vi "gaussian correlation time with pause.vi"() -> ()   [LabVIEW 2014]
uses:
  <vilib>/userdefined/High Color/IMAQdx.ctl
  <vilib>/Utility/file.llb/Write To Spreadsheet File (DBL).vi
  <vilib>/vision/driver/NI_Vision_Acquisition_Software.lvlib
panel:
  in  "Stimulus Duration (frames)":dbl
  in  "Pause Duration (frames)":dbl
  in  "Correlation Time (s)":dbl
  in  "Start Recording":bool
  in  "Max Voltage":dbl
  in  "Min Voltage":dbl
  in  "Frames":i32
  in  "Sigma":dbl
  in  "Offset Voltage":dbl
  out "Error":string
  out "Save Directory":path
  out "Buffer Number Out":u32
  out "Image":T1(plugin-control)
  in  "stop":bool
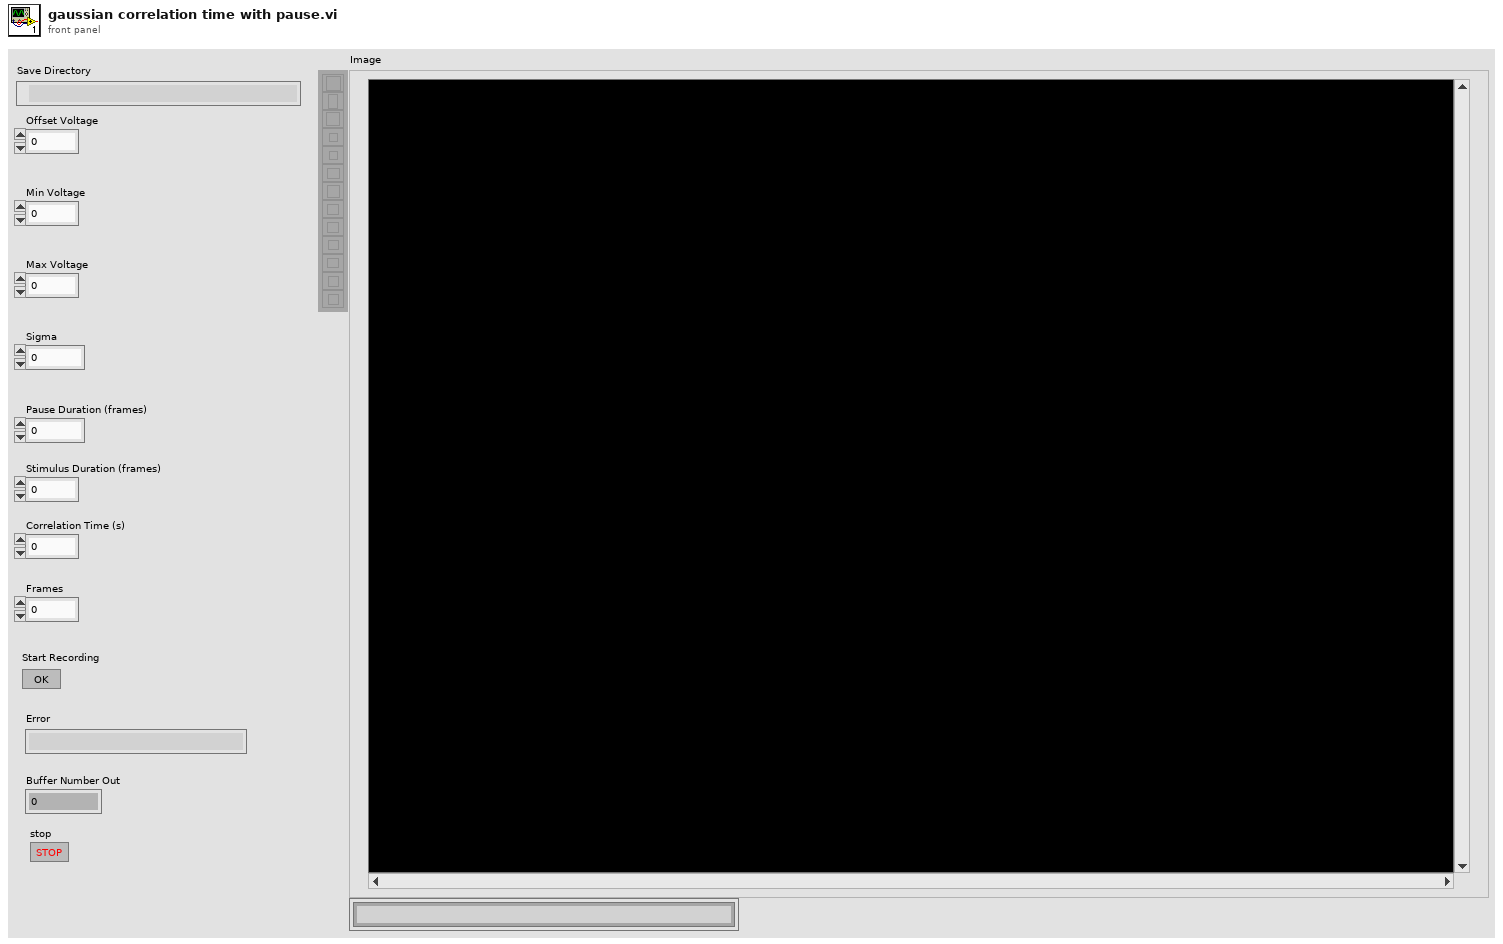
[diagram p1: front panel]
types:
  T1 = typedef "IMAQ Image.ctl" = refnum<image>
  T2 = typedef "IMAQdx.ctl" = refnum<k21>
  T3 = cluster{"Rows Per Strip":i32, "Photometric":i32, "Compression Type":i32}
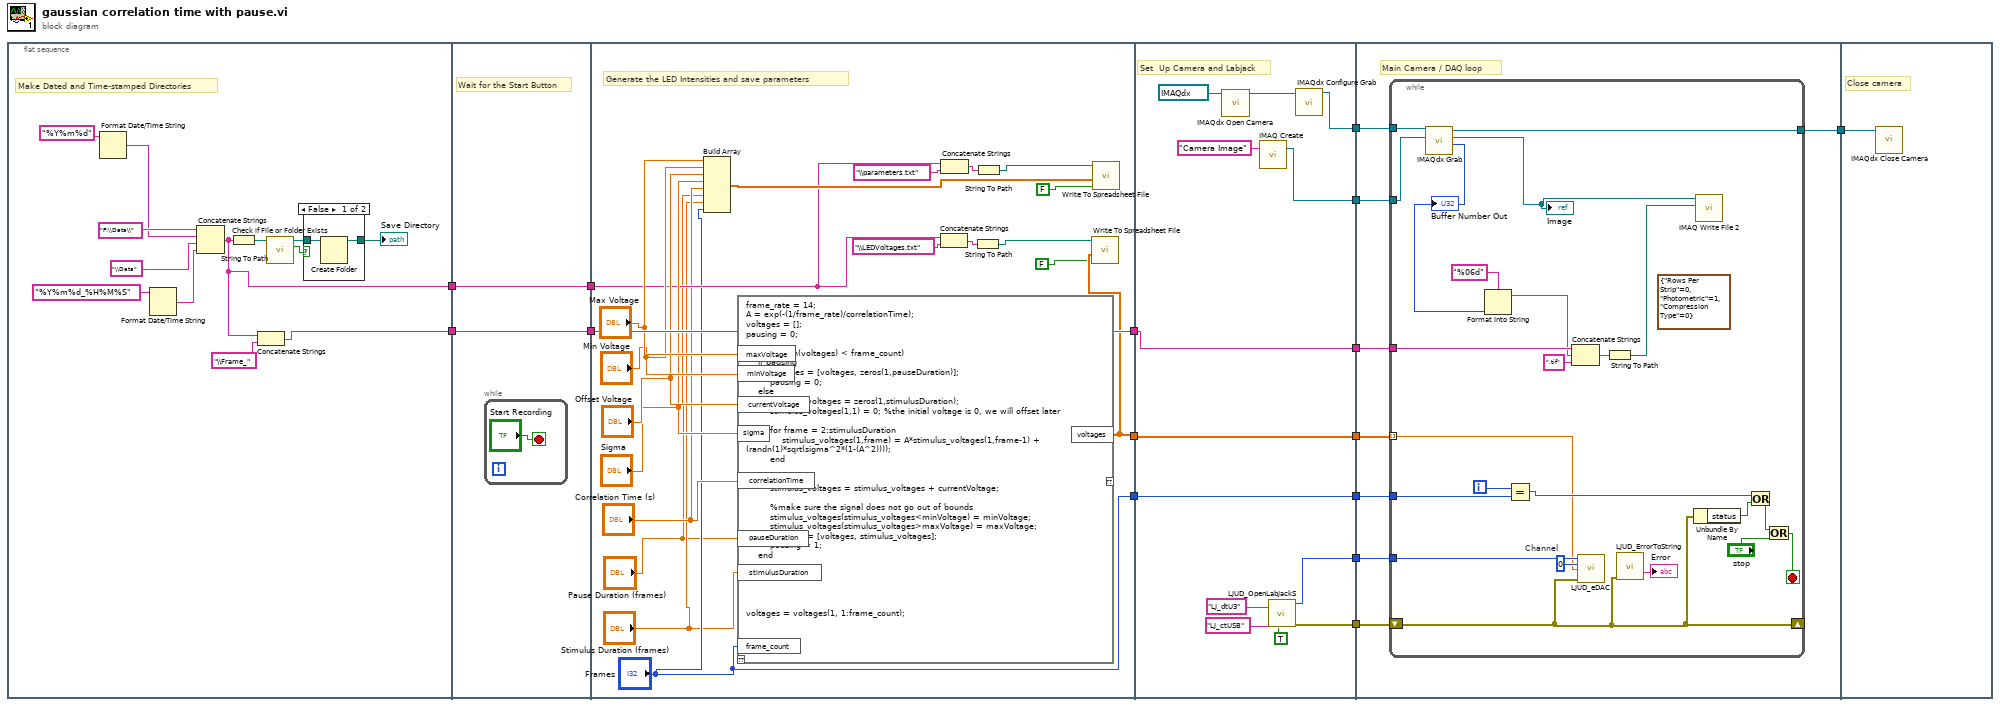
[diagram p0: block diagram]
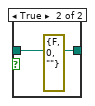
[diagram p2: hidden frame]
diagram:
  n1 = flat-sequence {
    tunnel: [w18] -> w4
    tunnel: [w16] -> w2
    tunnel: w4 -> [w33]
    tunnel: [w33] -> w3
    tunnel: w2 -> [w32]
    tunnel: [w32] -> w1
    tunnel: w3 -> [w52]
    tunnel: [w52] -> w9
    tunnel: [w50] -> w7
    tunnel: ["Frames"] -> w6
    tunnel: w1 -> [w39]
    tunnel: w9 -> [w62]
    tunnel: [w64] -> w15
    tunnel: [w63] -> w14
    tunnel: [w62] -> w13
    tunnel: [w58] -> w11
    tunnel: [w57] -> w10
    tunnel: [w56] -> w8
    tunnel: w7 -> [w56]
    tunnel: w6 -> [w55]
    tunnel: [w55] -> w5
    tunnel: w15 -> [w75]
    tunnel: w14 -> [w74]
    tunnel: w13 -> [w73]
    tunnel: [w72] -> w12
    tunnel: w11 -> [w71]
    tunnel: w10 -> [w70]
    tunnel: w8 -> [w69]
    tunnel: w5 -> [w68]
    tunnel: w12 -> [w99]
    frame #0 {
      # "Make Dated and Time-stamped Directories"
      n2 = Format Date/Time String(time format string (%c)="%Y%m%d") -> (date/time string=w19:string)  [unwired: 2 in]
      n3 = Format Date/Time String(time format string (%c)="%Y%m%d_%H%M%S") -> (date/time string=w23:string)  [unwired: 2 in]
      n4 = Concatenate Strings("F:\\Data\\", w19, "\\Data", w23) -> (w16:string)
      n5 = String To Path(string=w16) -> (path=w22:path)
      n6 = Concatenate Strings(w16, "\\Frame_") -> (w18:string)
      n7 = call <vilib>:"Check if File or Folder Exists.vi"("path"=w22) -> ("file or folder exists?"=w27:bool, "dup path"=w26:path)  [unwired: 8 in, 1 out]
      n8 = case shown="False" w27 {
        tunnel: [w29 w31] -> w21
        tunnel: w26 -> [w30 w31]
        frame False {
          n9 = Create Folder(path (use dialog)=w30) -> (created path=w29:path)  [unwired: 2 in, 2 out]
        }
        frame True {
          (unwired) errorcluster {"status"=FALSE, "code"=0, "source"=""} ("error out")
        }
      }
      "Save Directory" <- w21
    }
    frame #1 {
      # "Wait for the Start Button"
      n10 = while {
        stop <- "Start Recording" stop-if-true
      }
    }
    frame #2 {
      # "Generate the LED Intensities and save parameters"
      n11 = Build Array("Max Voltage", "Min Voltage", "Offset Voltage", "Sigma", "Correlation Time (s)", "Pause Duration (frames)", "Stimulus Duration (frames)", "Frames") -> (w40:dbl[])
      n12 = script code="frame_rate = 14;\nA = exp(-(1/frame_rate)/correlationTime);\nvoltages = [];\npausing = 0;\n\nwhile (length(voltages) < frame_count)\n    if pausing\n        voltages = [voltages, zeros(1,pauseDuration)];\n        pausing = 0;\n    else\n        stimulus_voltages = zeros(1,stimulusDuration);\n        stimulus_voltages(1,1) = 0; %the initial voltage is 0, we will offset later\n\n        for frame = 2:stimulusDuration\n            stimulus_voltages(1,frame) = A*stimulus_voltages(1,frame-1) + (randn(1)*sqrt(sigma^2*(1-(A^2))));\n        end\n\n        %offset\n        stimulus_voltages = stimulus_voltages + currentVoltage;\n\n        %make sure the signal does not go out of bounds\n        stimulus_voltages(stimulus_voltages<minVoltage) = minVoltage;\n        stimulus_voltages(stimulus_voltages>maxVoltage) = maxVoltage;\n        voltages = [voltages, stimulus_voltages];\n        pausing = 1;\n    end\n\nend\n\n\n\nvoltages = voltages(1, 1:frame_count);"("currentVoltage"="Offset Voltage", "frame_count"="Frames", "sigma"="Sigma", "minVoltage"="Min Voltage", "maxVoltage"="Max Voltage", "correlationTime"="Correlation Time (s)", "pauseDuration"="Pause Duration (frames)", "stimulusDuration"="Stimulus Duration (frames)") -> ("voltages"=w50:dbl[])  [unwired: 1 in, 1 out]
      n13 = Concatenate Strings(w39, "\\LEDVoltages.txt") -> (w54:string)
      n14 = Concatenate Strings(w39, "\\parameters.txt") -> (w44:string)
      n15 = String To Path(string=w54) -> (path=w53:path)
      n16 = String To Path(string=w44) -> (path=w43:path)
      n17 = call-poly <vilib>:"Write To Spreadsheet File.vi"("append to file? (new file:F)"=FALSE, "1D data"=w50, "file path (dialog if empty)"=w53) -> ()  [unwired: 5 in, 1 out]
      n18 = call-poly <vilib>:"Write To Spreadsheet File.vi"("append to file? (new file:F)"=FALSE, "1D data"=w40, "file path (dialog if empty)"=w43) -> ()  [unwired: 5 in, 1 out]
    }
    frame #3 {
      # "Set  Up Camera and Labjack"
      n19 = call <vilib>:"IMAQdx Open Camera.vi"("Session In"=T2 "cam0") -> ("Session Out"=w66:T2)  [unwired: 9 in, 1 out]
      n20 = call "IMAQ Create"("Image Name"="Camera Image") -> ("New Image"=w63:T1)  [unwired: 4 in, 1 out]
      n21 = call "LJUD_OpenLabJackS.vi"("FirstFound"=TRUE, "ConnectionType"="LJ_ctUSB", "DeviceType"="LJ_dtU3") -> ("error out"=w57:errorcluster, "Handle"=w58:i32)  [unwired: 6 in, 1 out]
      n22 = call <vilib>:"IMAQdx Configure Grab.vi"("Session In"=w66) -> ("Session Out"=w64:T2)  [unwired: 9 in, 1 out]
    }
    frame #4 {
      # "Main Camera / DAQ loop"
      n23 = while {
        tunnel: w75 -> [w98]
        tunnel: [w97] -> w72
        tunnel: w74 -> [w96]
        tunnel: w73 -> [w94]
        tunnel: w71 -> [w87]
        shift-right: [w84] -> _
        shift-left: w70 -> [w84]
        tunnel: w69 -> [w76] mode=indexing
        tunnel: w68 -> [w77]
        i -> [w78]
        stop <- w86 stop-if-true
        w83 = 0  # Channel
        (unwired) T3 {"Rows Per Strip"=0, "Photometric"=1, "Compression Type"=0} ("TIFF Options")
        n24 = call <vilib>:"IMAQdx Grab.vi"("Image In"=w96, "Session In"=w98) -> ("Buffer Number Out"=w90:u32, "Image Out"=w95:T1, "Session Out"=w97:T2)  [unwired: 6 in, 1 out]
        "Image" <- w95
        "Buffer Number Out" <- w90
        n25 = Format Into String(format string="%06d" ("string"), w90) -> (resulting string=w89:string)  [unwired: 2 in, 1 out]
        n26 = Equal?(x=w78, y=w77) -> (x = y?=w80:bool)
        n27 = Concatenate Strings(w94, w89, ".tif" ("string")) -> (w92:string)
        n28 = call "LJUD_eDAC.vi"("Handle In"=w87, "Channel"=w83, "Voltage"=w76, "error in"=w84) -> ()  [unwired: 10 in, 2 out]
        n29 = String To Path(string=w92) -> (path=w91:path)
        n30 = call "LJUD_ErrorToString.vi"("error in"=w84) -> ("String"=→"Error":string)  [unwired: 10 in]
        n31 = Unbundle By Name(w84) -> ("status"=w81:bool)
        n32 = call-poly "IMAQ Write File 2"("File Path"=w91, "Image"=w95) -> ()  [unwired: 8 in, 2 out]
        n33 = Or(x=w80, y=w81) -> (x .or. y?=w79:bool)
        n34 = Or(x=w79, y="stop") -> (x .or. y?=w86:bool)
      }
    }
    frame #5 {
      # "Close camera"
      n35 = call <vilib>:"IMAQdx Close Camera.vi"("Session In"=w99) -> ()  [unwired: 10 in, 1 out]
    }
  }
